vi "templates standard BODY data keys.vi"(9 "Template Keys":T1, 10 "HTM Keys":T1) -> (2 "HTM Keys":T1)   [LabVIEW 2011]
uses:
  Addons/internet/utils/keyedarr.llb/Keyed Array.ctl
  Addons/internet/utils/strutil.llb/Case Matching.ctl
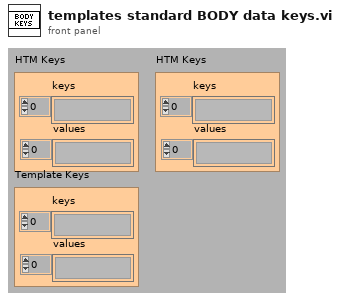
[diagram p1: front panel]
types:
  T1 = typedef "Keyed Array.ctl" = cluster{"keys":string[], "values":string[]}
  T2 = typedef "Case Matching.ctl" = enum16{"a != A", "a == A", "system"}
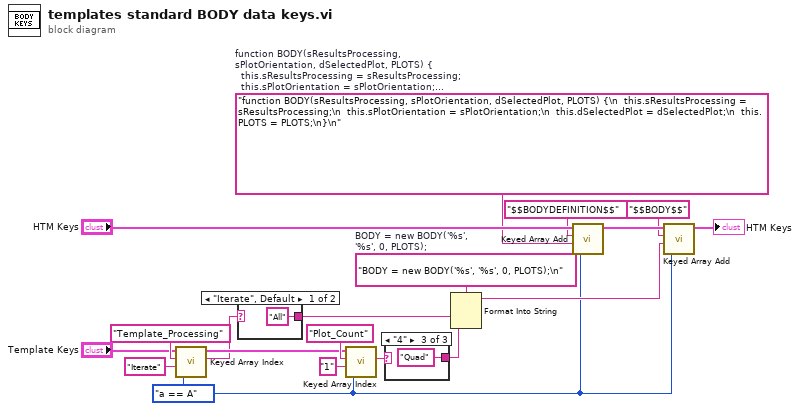
[diagram p0: block diagram]
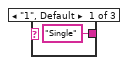
[diagram p3: hidden frame]
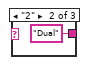
[diagram p4: hidden frame]
diagram:
  w5 = Case_Matching."a == A" ("case matching (sensitive)")
  w13 = "BODY = new BODY('%s', '%s', 0, PLOTS);\n"  # BODY = new BODY('%s', '%s', 0, PLOTS);
  w17 = "function BODY(sResultsProcessing, sPlotOrientation, dSelectedPlot, PLOTS) {\n  this.sResultsProcessing = sResultsProcessing;\n  this.sPlotOrientation = sPlotOrientation;\n  this.dSelectedPlot = dSelectedPlot;\n  this.PLOTS = PLOTS;\n}\n"  # function BODY(sResultsProcessing, sPlotOrientation, dSelectedPlot, PLOTS) {   this.sResultsProcessing = sResultsProcessing;   this.sPlotOrientation = sPlotOrientation;   this.dSelectedPlot = dSelectedPlot;   this.PLOTS = PLOTS; }
  n1 = call "Keyed Array Index.vi"("case matching (sensitive)"=w5, "default value"="Iterate" ("key"), "key"="Template_Processing", "array in"="Template Keys") -> ("value"=w2:string, "duplicate array"=w3:T1)  [unwired: 2 out]
  n2 = case shown="\"Iterate\", Default" w2 {
    selector: w2 -> [_ w21]
    tunnel: ["All" ("key") w21] -> w1
    frame "Iterate", Default {
    }
    frame "Most Recent" {
    }
  }
  n3 = call "Keyed Array Index.vi"("case matching (sensitive)"=w5, "default value"="1" ("key"), "key"="Plot_Count", "array in"=w3) -> ("value"=w10:string)  [unwired: 3 out]
  n4 = case shown="\"4\"" w10 {
    tunnel: ["Single" ("key") "Dual" ("key") "Quad" ("key")] -> w9
    frame "1", Default {
    }
    frame "2" {
    }
    frame "4" {
    }
  }
  n5 = Format Into String(format string=w13, w1, w9) -> (resulting string=w8:string)  [unwired: 2 in, 1 out]
  n6 = call "Keyed Array Add.vi"("case matching (sensitive)"=w5, "value"=w17, "key"="$$BODYDEFINITION$$", "array in"="HTM Keys") -> ("array out"=w16:T1)  [unwired: 3 out]
  n7 = call "Keyed Array Add.vi"("case matching (sensitive)"=w5, "value"=w8, "key"="$$BODY$$", "array in"=w16) -> ("array out"=→"HTM Keys":T1)  [unwired: 3 out]
